vi "信息流测试(子VI).vi"(11 "队列输入":refnum<queue>) -> (3 "簇":T1)   [LabVIEW 2019, in "test.lvlib"]
uses:
  SubVI/test.lvlib
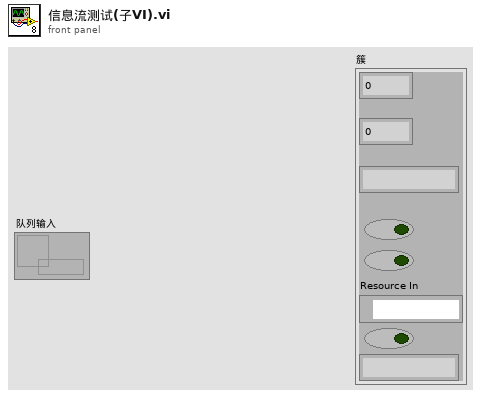
[diagram p1: front panel]
types:
  T1 = typedef "test.lvlib/控件 1.ctl" = cluster{i32, "数值 2":i32, "字符串":string, "布尔":bool, bool, "Resource In":refnum<visa-resource-name>, bool, string}
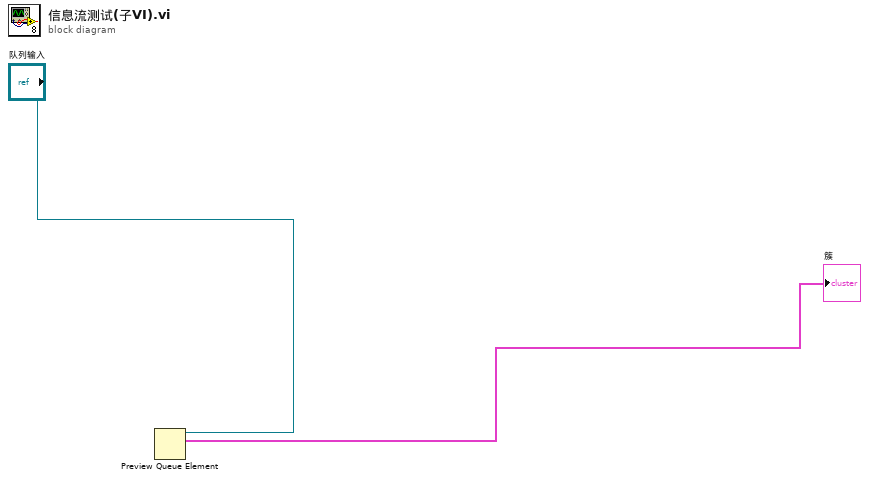
[diagram p0: block diagram]
diagram:
  n1 = Preview Queue Element(queue="队列输入") -> (element=→"簇":T1)  [unwired: 2 in, 3 out]
